vi "InputCoupleSet.vi"(0 "SR865 in":T2, 2 "InputCouple":T1 caption="Input couple" items=["AC", "DC"], 5 "error in":errorcluster) -> (14 "SR865 out":T2, 19 "error out":errorcluster)   [LabVIEW 2017]
uses:
  SR865.ctl
  InputCouple.ctl
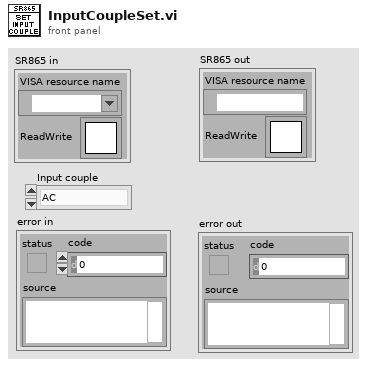
[diagram p1: front panel]
types:
  T1 = typedef "InputCouple.ctl" = u16
  T2 = typedef "SR865.ctl" = cluster{"VISA resource name":refnum<visa-resource-name>, "ReadWrite":T3}
  T3 = typedef "Semaphore RefNum" = refnum<k1>
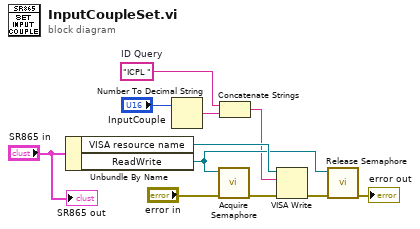
[diagram p0: block diagram]
diagram:
  w3 = "ICPL "  # ID Query
  n1 = Unbundle By Name("SR865 in") -> ("VISA resource name"=w10:refnum<visa-resource-name>, "ReadWrite"=w6:T3)
  n2 = Number To Decimal String(number="InputCouple") -> (decimal integer string=w2:string)  [unwired: 1 in]
  n3 = call <vilib>:"Acquire Semaphore.vi"("error in (no error)"="error in", "semaphore"=w6) -> ("error out"=w9:errorcluster)  [unwired: 3 in, 2 out]
  n4 = Concatenate Strings(w3, w2) -> (w1:string)
  n5 = VISA Write(VISA resource name=w10, write buffer=w1, error in (no error)=w9) -> (error out=w4:errorcluster)  [unwired: 2 out]
  n6 = call <vilib>:"Release Semaphore.vi"("error in (no error)"=w4, "semaphore"=w6) -> ("error out"=→"error out":errorcluster)  [unwired: 4 in, 1 out]
  "SR865 out" <- "SR865 in"
